vi "快速XY波形图.vi"() -> ()   [LabVIEW 2010]
uses:
  Instance           2 20Saved   快速XY Graph .vi
  Instance           4 20Saved   快速XY Graph .vi
  Instance           7 20Saved   快速XY Graph .vi
  Instance           6 20Saved   快速XY Graph .vi
  Instance           3 20Saved   快速XY Graph .vi
  Instance           5 20Saved   快速XY Graph .vi
  <vilib>/Analysis/NI_AALBase.lvlib
panel:
  out "XY Graph":cluster{"Y":dbl[], "Y":dbl[]}[](graph)
  out "XY Graph":cluster{"Y":dbl[], "Y":dbl[]}[](graph)
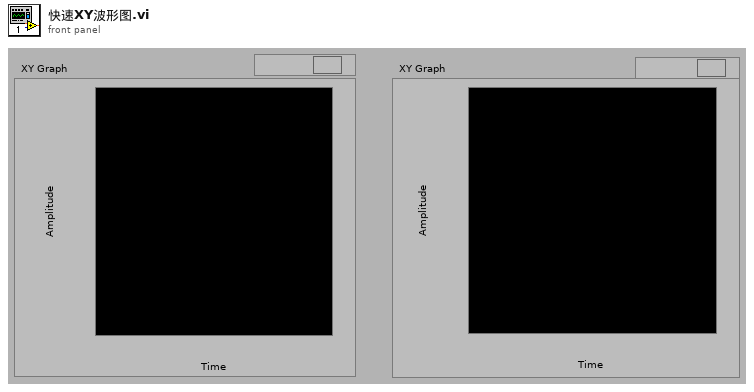
[diagram p1: front panel]
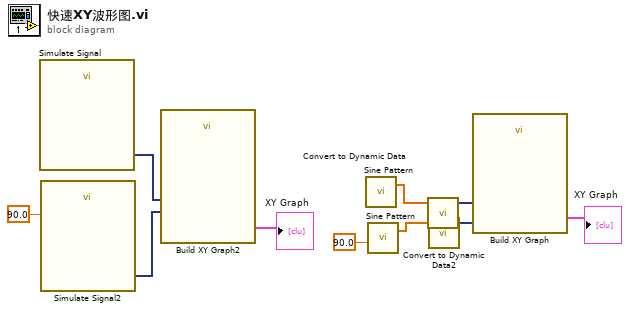
[diagram p0: block diagram]
diagram:
  n1 = call "Simulate Signal"() -> ("Sine"=w7:dynamicdata)  [unwired: 14 in, 1 out]
  n2 = call "Simulate Signal2"("Phase"=90.0) -> ("Sine"=w6:dynamicdata)  [unwired: 13 in, 1 out]
  n3 = call "Build XY Graph2"("Y Input"=w6, "X Input"=w7) -> ("XY Graph"=→"XY Graph":cluster{"Y":dbl[], "Y":dbl[]}[])  [unwired: 8 in, 1 out]
  n4 = call <vilib>:"Sine Pattern.vi"() -> ("Sinusoidal Pattern"=w10:dbl[])  [unwired: 4 in, 1 out]
  n5 = call <vilib>:"Sine Pattern.vi"("phase(degrees)"=90.0) -> ("Sinusoidal Pattern"=w9:dbl[])  [unwired: 3 in, 1 out]
  n6 = call "Convert to Dynamic Data"("Array"=w10) -> ("Dynamic Data Type"=w4:dynamicdata)  [unwired: 3 in]
  n7 = call "Convert to Dynamic Data2"("Array"=w9) -> ("Dynamic Data Type"=w3:dynamicdata)  [unwired: 3 in]
  n8 = call "Build XY Graph"("Y Input"=w3, "X Input"=w4) -> ("XY Graph"=→"XY Graph":cluster{"Y":dbl[], "Y":dbl[]}[])  [unwired: 8 in, 1 out]
